vi "New.vi"(0 "Topic URI":string, 5 "Notify result":bool, 7 "Arguments":string, 9 "ArgumentsKw":string, 11 "error in (no error)":errorcluster, 12 "Options":string) -> (4 "CallRequest (JSON) out":refnum<class "CallRequest (JSON).lvclass">, 6 "Notifier out":refnum<notifier>, 15 "error out":errorcluster)   [LabVIEW 2020, in "wamplv.lvlib" / "CallRequest (JSON).lvclass"]
uses:
  CallRequest (JSON).lvclass
  CallRequest (JSON).lvclass/CallRequest (JSON).ctl
  f7d0075e-672a-4c76-bb20-5e1e6ee839c4.vi
  WAMP Client/API/TypeDefs/Error or abort detail (JSON).ctl
  wamplv.lvlib
  WAMP Client/API/TypeDefs/RESULT payload (JSON).ctl
  WAMP Client/WAMP Client.lvclass
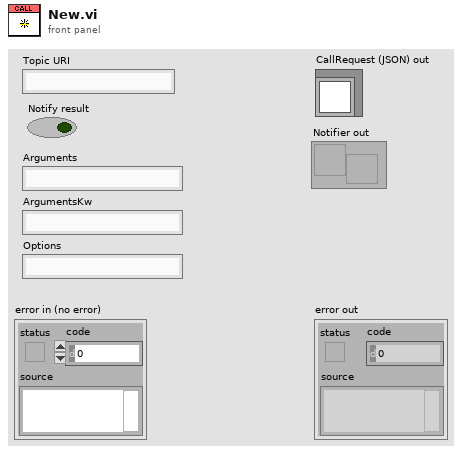
[diagram p1: front panel]
types:
  T1 = typedef "wamplv.lvlib/WAMP Client.lvclass/RESULT payload (JSON).ctl" = cluster{"Topic":string, "Arguments Payload":string, "ArgumentKw Payload":string, "Details":string, "Error/Abort details (JSON)":T2}
  T2 = typedef "wamplv.lvlib/Error or abort detail (JSON).ctl" = cluster{"Error URI":string, "Error Arguments":string, "Error ArgumentKw":string, "Error Details":string, "Associated LabVIEW Error":errorcluster}
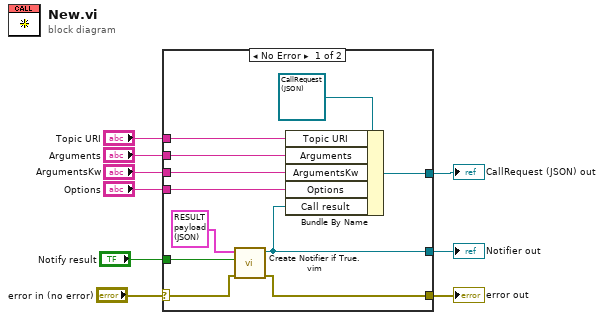
[diagram p0: block diagram]
diagram:
  n1 = case shown="No Error" "error in (no error)" {
    selector: "error in (no error)" -> [w13 w21]
    tunnel: [w12 w21] -> w8
    tunnel: "Topic URI" -> [w19 _]
    tunnel: "Arguments" -> [w18 _]
    tunnel: "ArgumentsKw" -> [w17 _]
    tunnel: "Options" -> [w16 _]
    tunnel: "Notify result" -> [w14 _]
    tunnel: [w11 _] -> w2
    tunnel: [w10 _] -> w1
    frame No Error {
      n2 = call "Create Notifier if True.vim"("error in (no error)"=w13, "Boolean"=w14, "RESULT Payload"=T1 {"Topic"="", "Arguments Payload"="", "ArgumentKw Payload"="", "Details"="[]", "Error/Abort details (JSON)"={"Error URI"="", "Error Arguments"="", "Error ArgumentKw"="{}", "Error Details"="{}", "Associated LabVIEW Error"={"status"=FALSE, "code"=0, "source"=""}}}) -> ("error out"=w12:errorcluster, "Notifier out"=w11:refnum<notifier>)  [unwired: 7 in]
      n3 = Bundle By Name(cluster=refnum<class "CallRequest (JSON).lvclass"> refnum ("wamplv.lvlib:CallRequest (JSON).lvclass"), "Topic URI"=w19, "Arguments"=w18, "ArgumentsKw"=w17, "Options"=w16, "Call result"=w11) -> (w10:refnum<class "CallRequest (JSON).lvclass">)
    }
    frame Error {
    }
  }
  "error out" <- w8
  "CallRequest (JSON) out" <- w1
  "Notifier out" <- w2
